vi "Crosspoint_y.vi"(0 "Discharge X channels?":bool=TRUE, 1 "Y Channel Ground":string="y1", 2 "Array":string[](array[combo])=["NC", "NC", "NC", "NC", "NC", "NC", "NC", "NC"], 3 "Discharge Y Channels?":bool=TRUE, 4 "X Channel Ground":string="x12") -> ()   [LabVIEW 2010]
panel:
  in  "IVI Option String":string="Simulate=0,RangeCheck=1,QueryInstrStatus=0,Cache=1,DriverSetup=Model:40-726-511;"
  in  "VISA Resource Name":string="PXI9::13::INSTR"
  # "y1"
  # "y2"
  # "y3"
  # "y4"
  # "y5"
  # "y6"
  # "y7"
  # "y8"
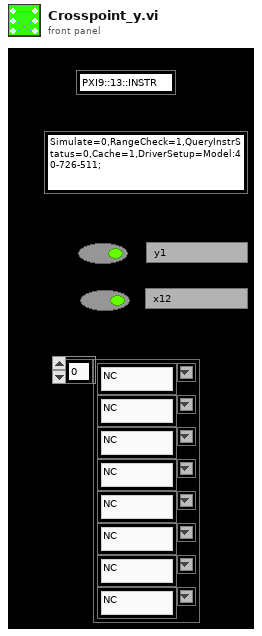
[diagram p1: front panel]
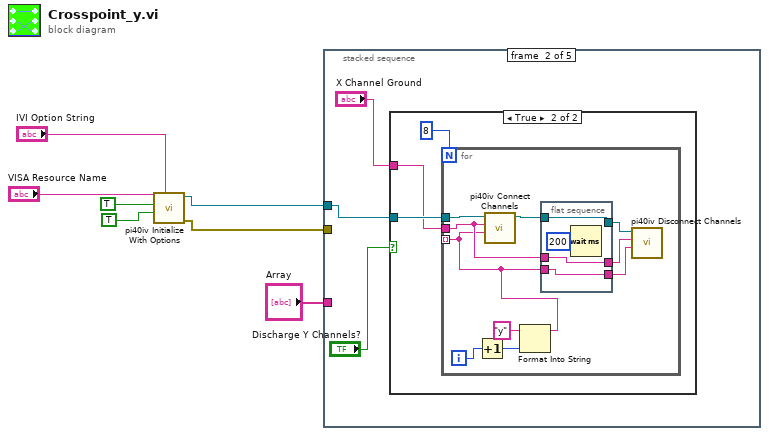
[diagram p0: block diagram]
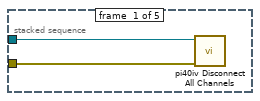
[diagram p2: hidden frame]
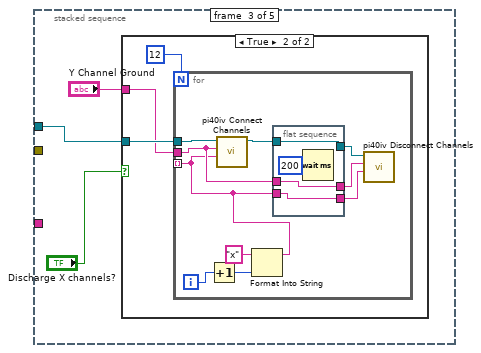
[diagram p4: hidden frame]
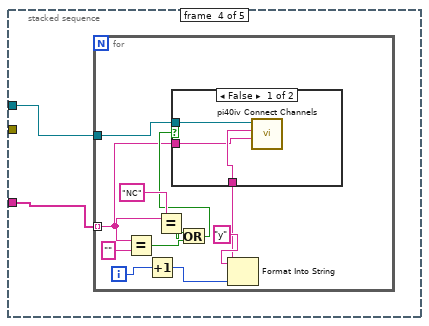
[diagram p6: hidden frame]
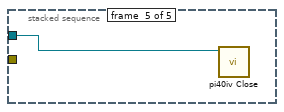
[diagram p8: hidden frame]
diagram:
  n1 = call <instrlib>:"pi40iv Initialize With Options.vi"("option string"="IVI Option String", "reset device"=TRUE, "id query"=TRUE, "resource name"="VISA Resource Name") -> ("error out"=w2:errorcluster, "instrument handle out"=w3:refnum<k15>)  [unwired: 6 in]
  n2 = stacked-sequence {
    tunnel: w3 -> [w9 w10 w32 w51 w66]
    tunnel: w2 -> [w8 _ _ _ _]
    tunnel: "Array" -> [_ _ _ w50 _]
    frame #0 {
      n3 = call <instrlib>:"pi40iv Disconnect All Channels.vi"("error in (no error)"=w8, "instrument handle"=w9) -> ()  [unwired: 8 in, 2 out]
    }
    frame #1 {
      n4 = case shown="True" "Discharge Y Channels?" {
        tunnel: w10 -> [_ w15]
        tunnel: "X Channel Ground" -> [_ w14]
        frame False {
        }
        frame True {
          n5 = for {
            N: 8 -> [_]
            tunnel: w15 -> [w25]
            tunnel: w14 -> [w22]
            tunnel: [w17] -> _ mode=indexing
            i -> [w18]
            n6 = Increment(x=w18) -> (x+1=w16:i32)
            n7 = Format Into String(initial string="y", w16) -> (resulting string=w17:string)  [unwired: 2 in, 1 out]
            n8 = call <instrlib>:"pi40iv Connect Channels.vi"("channel 2"=w17, "channel 1"=w22, "instrument handle"=w25) -> ("instrument handle out"=w24:refnum<k15>)  [unwired: 7 in, 1 out]
            n9 = flat-sequence {
              tunnel: w24 -> [w29]
              tunnel: [w29] -> w23
              tunnel: w22 -> [w27]
              tunnel: [w27] -> w21
              tunnel: w17 -> [w26]
              tunnel: [w26] -> w20
              frame #0 {
                n10 = Wait (ms)(milliseconds to wait=u32 200) -> ()  [unwired: 1 out]
              }
            }
            n11 = call <instrlib>:"pi40iv Disconnect Channels.vi"("channel 2"=w20, "channel 1"=w21, "instrument handle"=w23) -> ()  [unwired: 7 in, 2 out]
          }
        }
      }
    }
    frame #2 {
      n12 = case shown="True" "Discharge X channels?" {
        tunnel: w32 -> [_ w35]
        tunnel: "Y Channel Ground" -> [_ w34]
        frame False {
        }
        frame True {
          n13 = for {
            N: 12 -> [_]
            tunnel: w35 -> [w45]
            tunnel: w34 -> [w42]
            tunnel: [w37] -> _ mode=indexing
            i -> [w38]
            n14 = Increment(x=w38) -> (x+1=w36:i32)
            n15 = Format Into String(initial string="x", w36) -> (resulting string=w37:string)  [unwired: 2 in, 1 out]
            n16 = call <instrlib>:"pi40iv Connect Channels.vi"("channel 2"=w37, "channel 1"=w42, "instrument handle"=w45) -> ("instrument handle out"=w44:refnum<k15>)  [unwired: 7 in, 1 out]
            n17 = flat-sequence {
              tunnel: w44 -> [w49]
              tunnel: [w49] -> w43
              tunnel: w42 -> [w47]
              tunnel: [w47] -> w41
              tunnel: w37 -> [w46]
              tunnel: [w46] -> w40
              frame #0 {
                n18 = Wait (ms)(milliseconds to wait=u32 200) -> ()  [unwired: 1 out]
              }
            }
            n19 = call <instrlib>:"pi40iv Disconnect Channels.vi"("channel 2"=w40, "channel 1"=w41, "instrument handle"=w43) -> ()  [unwired: 7 in, 2 out]
          }
        }
      }
    }
    frame #3 {
      n20 = for {
        tunnel: w51 -> [w62]
        tunnel: w50 -> [w54] mode=indexing
        i -> [w61]
        n21 = Equal?(x=w54, y="") -> (x = y?=w53:bool)
        n22 = Increment(x=w61) -> (x+1=w59:i32)
        n23 = Equal?(x=w54, y="NC") -> (x = y?=w56:bool)
        n24 = Or(x=w56, y=w53) -> (x .or. y?=w55:bool)
        n25 = Format Into String(initial string="y" ("string"), w59) -> (resulting string=w58:string)  [unwired: 2 in, 1 out]
        n26 = case shown="False" w55 {
          tunnel: w62 -> [w65 _]
          tunnel: w58 -> [w64 _]
          tunnel: w54 -> [w63 _]
          frame False {
            n27 = call <instrlib>:"pi40iv Connect Channels.vi"("channel 2"=w63, "channel 1"=w64, "instrument handle"=w65) -> ()  [unwired: 7 in, 2 out]
          }
          frame True {
          }
        }
      }
    }
    frame #4 {
      n28 = call <instrlib>:"pi40iv Close.vi"("instrument handle"=w66) -> ()  [unwired: 10 in, 1 out]
    }
  }
